vi "Get_System_Boolean_Values.vi"(2 "error in":errorcluster, 3 "Data in":T1) -> (0 "error out":errorcluster, 1 "Data out":T1)   [LabVIEW 2015]
uses:
  Type_Defs/Data.ctl
  Type_Defs/Diagnostics.ctl
  Type_Defs/Systems.ctl
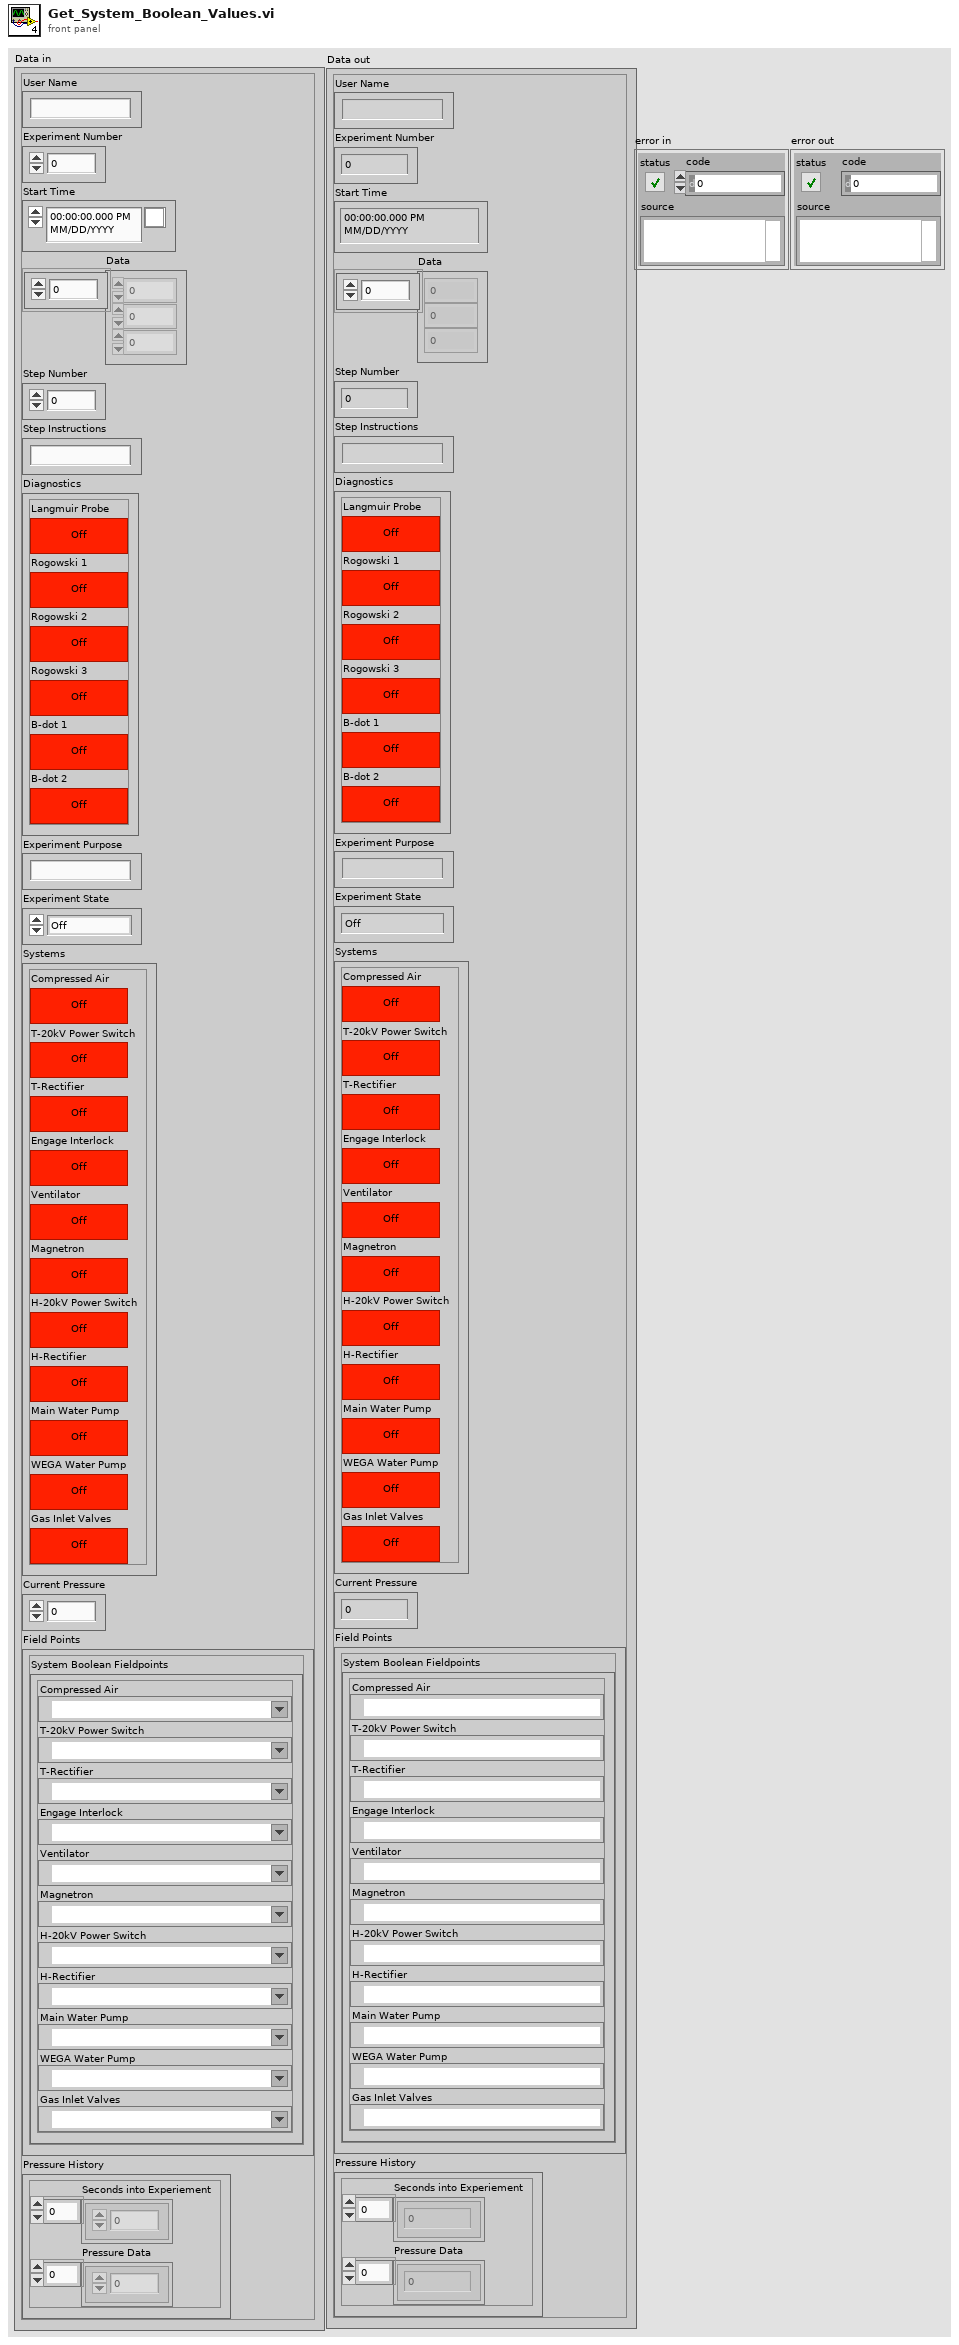
[diagram p1: front panel]
types:
  T1 = typedef "Data.ctl" = cluster{"User Name":string, "Experiment Number":i32, "Start Time":timestamp, "Data":dbl[], "Step Number":i32, "Step Instructions":string, "Diagnostics":T2, "Experiment Purpose":string, "Experiment State":enum16{"Off", "Setting Up", "Ready", "In Progress", "Shutting Down"}, "Systems":T3, "Current Pressure":dbl, "Field Points":cluster{"System Boolean Fieldpoints":cluster{"Compressed Air":refnum<k21>, "T-20kV Power Switch":refnum<k21>, "T-Rectifier":refnum<k21>, "Engage Interlock":refnum<k21>, "Ventilator":refnum<k21>, "Magnetron":refnum<k21>, "H-20kV Power Switch":refnum<k21>, "H-Rectifier":refnum<k21>, "Main Water Pump":refnum<k21>, "WEGA Water Pump":refnum<k21>, "Gas Inlet Valves":refnum<k21>}}, "Pressure History":cluster{"Seconds into Experiement":i32[], "Pressure Data":dbl[]}}
  T2 = typedef "Diagnostics.ctl" = cluster{"Langmuir Probe":bool, "Rogowski 1":bool, "Rogowski 2":bool, "Rogowski 3":bool, "B-dot 1":bool, "B-dot 2":bool}
  T3 = typedef "Systems.ctl" = cluster{"Compressed Air":bool, "T-20kV Power Switch":bool, "T-Rectifier":bool, "Engage Interlock":bool, "Ventilator":bool, "Magnetron":bool, "H-20kV Power Switch":bool, "H-Rectifier":bool, "Main Water Pump":bool, "WEGA Water Pump":bool, "Gas Inlet Valves":bool}
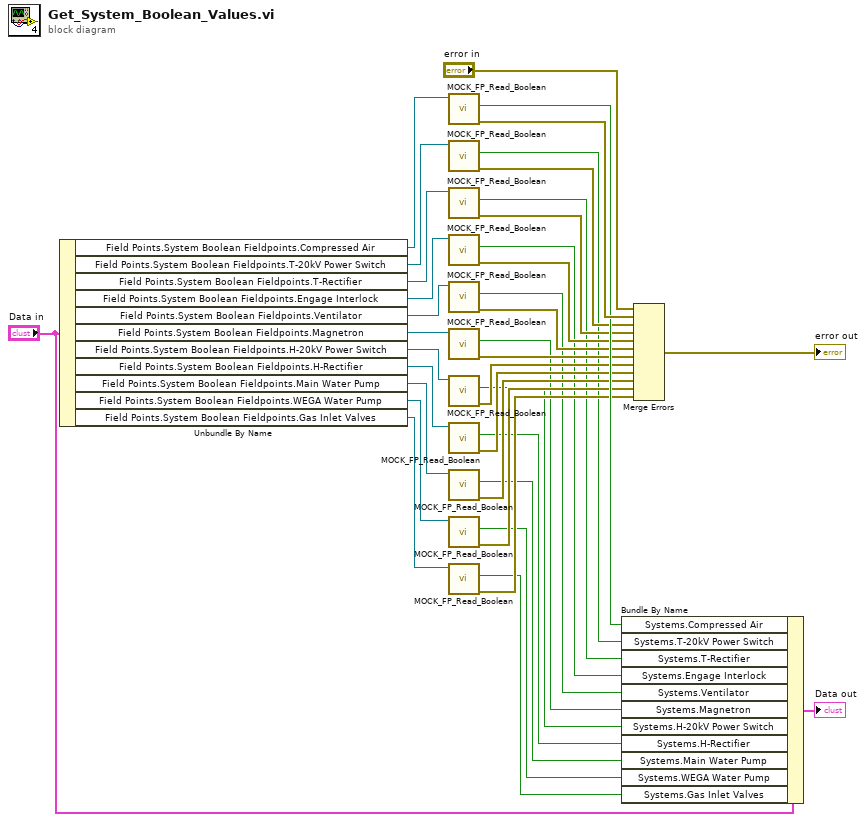
[diagram p0: block diagram]
diagram:
  n1 = Unbundle By Name("Data in") -> ("Field Points.System Boolean Fieldpoints.Compressed Air"=w37:refnum<k21>, "Field Points.System Boolean Fieldpoints.T-20kV Power Switch"=w32:refnum<k21>, "Field Points.System Boolean Fieldpoints.T-Rectifier"=w31:refnum<k21>, "Field Points.System Boolean Fieldpoints.Engage Interlock"=w30:refnum<k21>, "Field Points.System Boolean Fieldpoints.Ventilator"=w29:refnum<k21>, "Field Points.System Boolean Fieldpoints.Magnetron"=w28:refnum<k21>, "Field Points.System Boolean Fieldpoints.H-20kV Power Switch"=w27:refnum<k21>, "Field Points.System Boolean Fieldpoints.H-Rectifier"=w26:refnum<k21>, "Field Points.System Boolean Fieldpoints.Main Water Pump"=w25:refnum<k21>, "Field Points.System Boolean Fieldpoints.WEGA Water Pump"=w24:refnum<k21>, "Field Points.System Boolean Fieldpoints.Gas Inlet Valves"=w23:refnum<k21>)
  n2 = call "MOCK_FP_Read_Boolean.vi"("FieldPoint IO Point In"=w37) -> ("error out"=w34:errorcluster, "Boolean"=w33:bool)  [unwired: 7 in, 2 out]
  n3 = call "MOCK_FP_Read_Boolean.vi"("FieldPoint IO Point In"=w32) -> ("error out"=w22:errorcluster, "Boolean"=w11:bool)  [unwired: 7 in, 2 out]
  n4 = call "MOCK_FP_Read_Boolean.vi"("FieldPoint IO Point In"=w31) -> ("error out"=w21:errorcluster, "Boolean"=w10:bool)  [unwired: 7 in, 2 out]
  n5 = call "MOCK_FP_Read_Boolean.vi"("FieldPoint IO Point In"=w30) -> ("error out"=w20:errorcluster, "Boolean"=w9:bool)  [unwired: 7 in, 2 out]
  n6 = call "MOCK_FP_Read_Boolean.vi"("FieldPoint IO Point In"=w29) -> ("error out"=w19:errorcluster, "Boolean"=w8:bool)  [unwired: 7 in, 2 out]
  n7 = call "MOCK_FP_Read_Boolean.vi"("FieldPoint IO Point In"=w28) -> ("error out"=w18:errorcluster, "Boolean"=w7:bool)  [unwired: 7 in, 2 out]
  n8 = call "MOCK_FP_Read_Boolean.vi"("FieldPoint IO Point In"=w27) -> ("error out"=w17:errorcluster, "Boolean"=w5:bool)  [unwired: 7 in, 2 out]
  n9 = call "MOCK_FP_Read_Boolean.vi"("FieldPoint IO Point In"=w26) -> ("error out"=w16:errorcluster, "Boolean"=w4:bool)  [unwired: 7 in, 2 out]
  n10 = call "MOCK_FP_Read_Boolean.vi"("FieldPoint IO Point In"=w25) -> ("error out"=w15:errorcluster, "Boolean"=w3:bool)  [unwired: 7 in, 2 out]
  n11 = call "MOCK_FP_Read_Boolean.vi"("FieldPoint IO Point In"=w24) -> ("error out"=w14:errorcluster, "Boolean"=w2:bool)  [unwired: 7 in, 2 out]
  n12 = call "MOCK_FP_Read_Boolean.vi"("FieldPoint IO Point In"=w23) -> ("error out"=w13:errorcluster, "Boolean"=w1:bool)  [unwired: 7 in, 2 out]
  n13 = Bundle By Name(cluster="Data in", "Systems.Compressed Air"=w33, "Systems.T-20kV Power Switch"=w11, "Systems.T-Rectifier"=w10, "Systems.Engage Interlock"=w9, "Systems.Ventilator"=w8, "Systems.Magnetron"=w7, "Systems.H-20kV Power Switch"=w5, "Systems.H-Rectifier"=w4, "Systems.Main Water Pump"=w3, "Systems.WEGA Water Pump"=w2, "Systems.Gas Inlet Valves"=w1) -> (→"Data out":T1)
  n14 = Merge Errors("error in", w34, w22, w21, w20, w19, w18, w17, w16, w15, w14, w13) -> (→"error out":errorcluster)
